vi "Display.vi"(8 "error in":errorcluster, 11 "Plain - Three Button in":refnum<class "Plain - Three Button.lvclass">) -> (0 "error out":errorcluster, 3 "Plain - Three Button out":refnum<class "Plain - Three Button.lvclass">)   [LabVIEW 2021, in "Pop-Up.lvlib" / "Plain - Three Button.lvclass"]
doc: "This is the override method required for each child of the pop up class. It is the pop up that will display to the user.\n\nTo extend this function, create a child class of the pop up class. Then create an override method for this VI. <b>Display.vi</b> is a protected function, therefore it cannot be called in a main application. This VI must be called by a caller function. See one of the standard pop-ups for a setup example.\n\n<b>Code Developed By:</b> +\nDaniel Coons +\nhttps://github.com/danielcoons/tsc-pop-up"
uses:
  Plain - Three Button.lvclass
  C:/Development/Open Source/tsc-pop-up/Popup/Popup.lvclass
  C:/Development/Open Source/tsc-pop-up/Plain/Plain Parent.lvclass
  Popup/Popup.lvclass/Popup.ctl
  Plain Parent.lvclass/Plain Parent.ctl
  Plain - Three Button.lvclass/Plain - Three Button.ctl
  Popup/Data Member Access/Read Theme.vi
  Get Transparent buttons.vi
  Get Dialog Title.vi
  Get Action 1 Text.vi
  Get Action 2 Text.vi
  Get Action 3 Text.vi
  Theme/Theme.lvclass
  Popup/Popup.lvclass
  user32.dll
panel:
  in  "action 3":bool
  in  "action 2":bool
  out "dialog title":string
  out "message":string
  in  "action 1":bool
  # "This VI displays the popup"
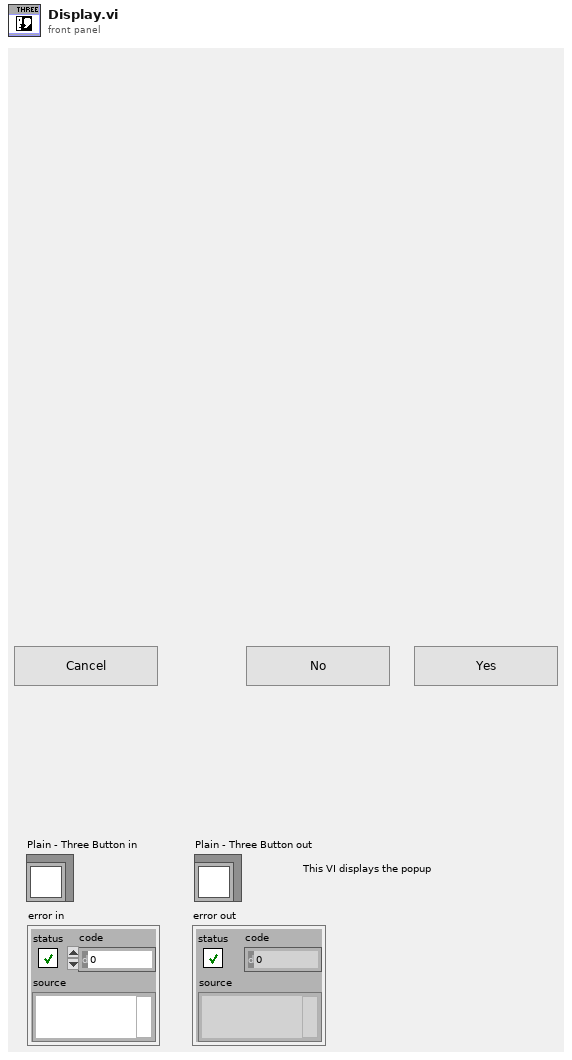
[diagram p1: front panel]
types:
  T1 = typedef "LVRectTypeDef.ctl" = cluster{"Left":i16, "Top":i16, "Right":i16, "Bottom":i16}
  T2 = typedef "LVPointTypeDef.ctl" = cluster{"Horizontal":i16, "Vertical":i16}
  T3 = typedef "LVPoint32TypeDef.ctl" = cluster{"Horizontal":i32, "Vertical":i32}
  T4 = typedef "LVPositionTypeDef.ctl" = cluster{"Left":i32, "Top":i32}
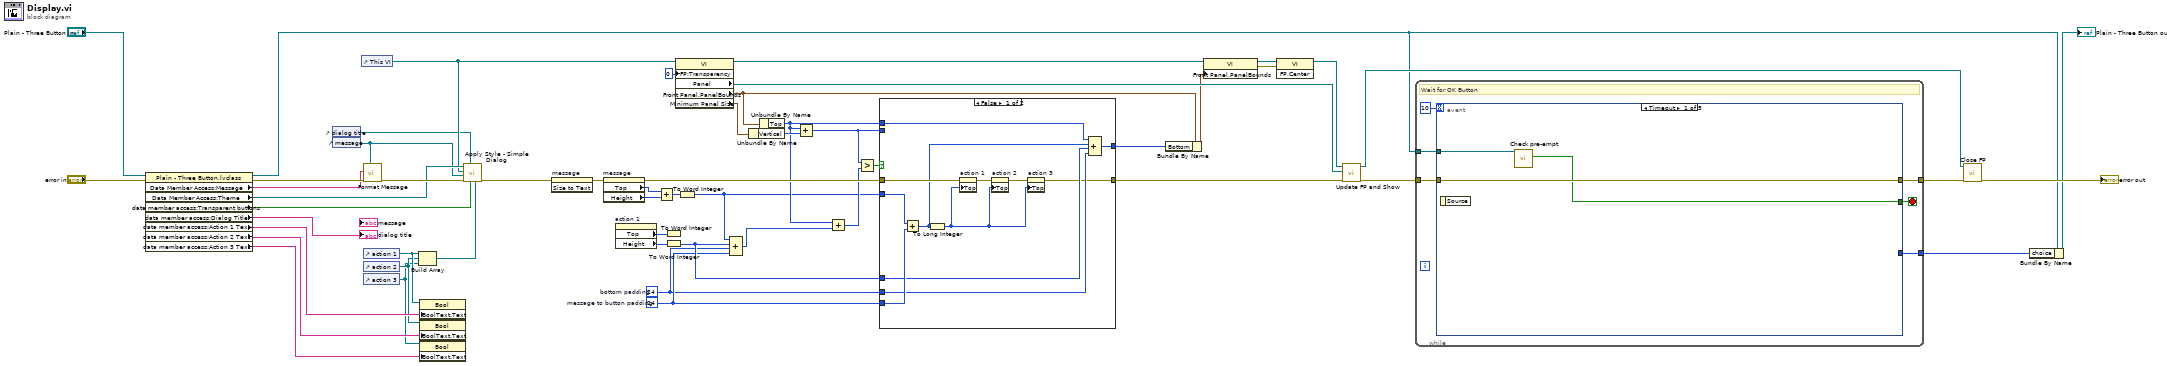
[diagram p0: block diagram]
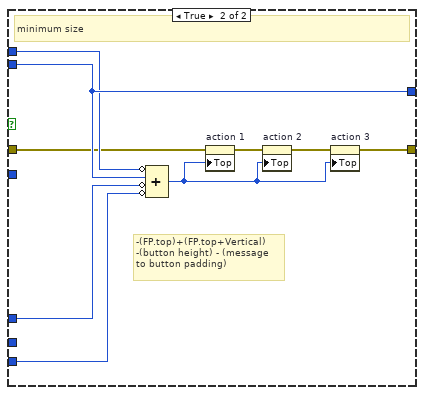
[diagram p2: hidden frame]
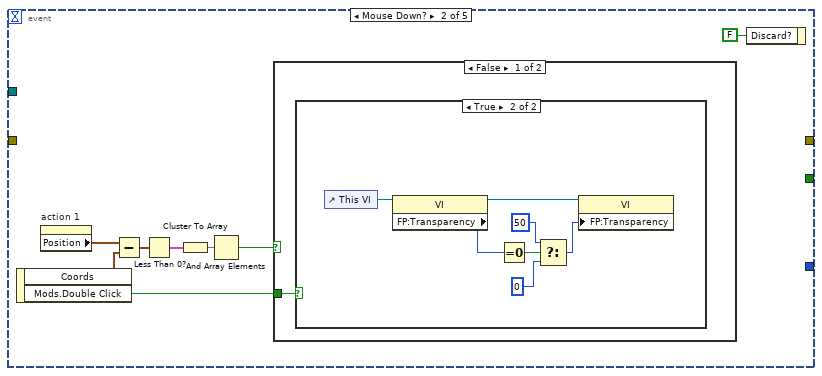
[diagram p3: hidden frame]
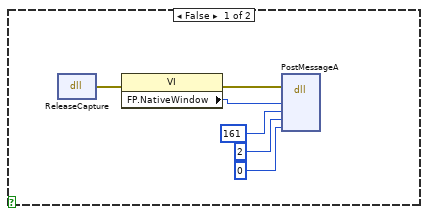
[diagram p4: hidden frame]
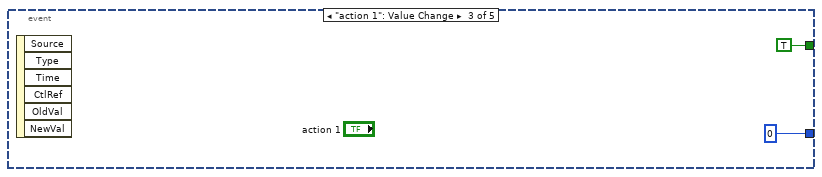
[diagram p6: hidden frame]
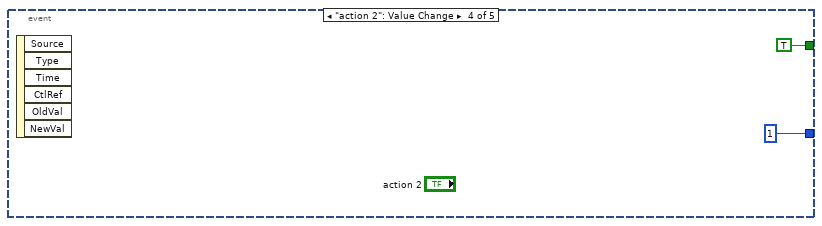
[diagram p7: hidden frame]
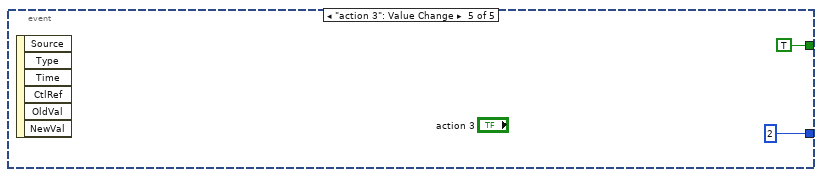
[diagram p8: hidden frame]
diagram:
  w26 = i16 24  # message to button padding
  w24 = i16 24  # bottom padding
  n1 = property class="Plain - Three Button.lvclass"(reference="Plain - Three Button in", error in="error in") -> (reference out=w2:refnum<class "Plain - Three Button.lvclass">, error out=w49:errorcluster, "Data Member Access:Message"=w45:string, "Data Member Access:Theme"=w18:refnum<class "Theme.lvclass">, "data member access:Transparent buttons"=w1:bool, "data member access:Dialog Title"=→"dialog title":string, "data member access:Action 1 Text"=w13:string, "data member access:Action 2 Text"=w12:string, "data member access:Action 3 Text"=w9:string)
  n2 = control-ref of="dialog title"() -> (w5:refnum<vi>)
  n3 = control-ref of="message"() -> (w6:refnum<vi>)
  n4 = control-ref of="This VI"() -> (w17:refnum<vi>)
  n5 = call "Format Message.vi"("formatted string"=w6, "error in"=w49, "String Input"=w45) -> ("error out"=w20:errorcluster)  [unwired: 7 in, 1 out]
  n6 = control-ref of="action 1"() -> (w14:refnum<vi>)
  n7 = control-ref of="action 2"() -> (w11:refnum<vi>)
  n8 = control-ref of="action 3"() -> (w10:refnum<vi>)
  n9 = Build Array(w14, w11, w10) -> (w16:refnum<vi>[])
  n10 = property class="Bool"(reference=w14, "BoolText.Text"=w13) -> ()  [unwired: 1 in, 2 out]
  n11 = property class="Bool"(reference=w11, "BoolText.Text"=w12) -> ()  [unwired: 1 in, 2 out]
  n12 = property class="Bool"(reference=w10, "BoolText.Text"=w9) -> ()  [unwired: 1 in, 2 out]
  n13 = call "Apply Style - Simple Dialog.vi"("button refs"=w16, "keep transparent buttons?"=w1, "title ref"=w5, "error in"=w20, "message ref"=w6, "pop up ref"=w17, "Theme in"=w18) -> ("error out"=w19:errorcluster)  [unwired: 3 in, 1 out]
  n14 = invoke on="message" class="Str" method="Size to Text"(error in=w19) -> (error out=w48:errorcluster)  [unwired: 2 in, 2 out]
  n15 = property on="message" class="Str"(error in=w48) -> (error out=w29:errorcluster, "Top"=w40:i32, "Height"=w39:u32)  [unwired: 1 in, 1 out]
  n16 = property on="action 1" class="Bool"() -> ("Top"=w42:i32, "Height"=w41:u32)  [unwired: 2 in, 2 out]
  n17 = Add(x=w40, y=w39) -> (x+y=w38:u32)
  n18 = To Word Integer(number=w42) -> ()  [unwired: 1 out]
  n19 = To Word Integer(number=w41) -> (16bit integer=w27:i16)
  n20 = property class="VI"(reference=w17, "FP:Transparency"=u8 0 ("Front Panel Window:Transparency")) -> (reference out=w44:refnum<vi>, "Panel"=w43:refnum<vi>, "Front Panel.PanelBounds"=w34:T1, "Minimum Panel Size"=w37:T2)  [unwired: 1 in, 1 out]
  n21 = To Word Integer(number=w38) -> (16bit integer=w3:i16)
  n22 = Compound Arithmetic op=ADD(w3, w27, w24, w26) -> (w4:i16)
  n23 = Unbundle By Name(w37) -> ("Vertical"=w36:i16)
  n24 = Unbundle By Name(w34) -> ("Top"=w21:i16)
  n25 = Add(x=w21, y=w36) -> (x+y=w22:i16)
  n26 = Add(x=w21, y=w4) -> (x+y=w23:i16)
  n27 = Greater?(x=w22, y=w23) -> (0:w30:bool)
  n28 = case shown="False" w30 {
    tunnel: [w65 w75] -> w25
    tunnel: w22 -> [_ w75]
    tunnel: w3 -> [w66 _]
    tunnel: w21 -> [w59 w74]
    tunnel: w29 -> [w64 w73]
    tunnel: [w56 w67] -> w28
    tunnel: w27 -> [w61 w72]
    tunnel: w26 -> [w63 w71]
    tunnel: w24 -> [w62 _]
    frame False {
      n29 = Add(x=w66, y=w63) -> (x+y=w60:i16)
      n30 = To Long Integer(number=w60) -> (32bit integer=w55:i32)
      n31 = property on="action 1" class="Bool"(error in=w64, "Top"=w55) -> (error out=w58:errorcluster)  [unwired: 1 in, 1 out]
      n32 = property on="action 2" class="Bool"(error in=w58, "Top"=w55) -> (error out=w57:errorcluster)  [unwired: 1 in, 1 out]
      n33 = property on="action 3" class="Bool"(error in=w57, "Top"=w55) -> (error out=w56:errorcluster)  [unwired: 1 in, 1 out]
      n34 = Compound Arithmetic op=ADD(w59, w60, w61, w62) -> (w65:i16)
    }
    frame True {
      # "-(FP.top)+(FP.top+Vertical)\n-(button height) - (message\nto button padding)"
      # "minimum size"
      n35 = Compound Arithmetic op=ADD(invert w74, w75, invert w72, invert w71) -> (w68:i16)
      n36 = property on="action 1" class="Bool"(error in=w73, "Top"=w68) -> (error out=w70:errorcluster)  [unwired: 1 in, 1 out]
      n37 = property on="action 2" class="Bool"(error in=w70, "Top"=w68) -> (error out=w69:errorcluster)  [unwired: 1 in, 1 out]
      n38 = property on="action 3" class="Bool"(error in=w69, "Top"=w68) -> (error out=w67:errorcluster)  [unwired: 1 in, 1 out]
    }
  }
  n39 = Bundle By Name(cluster=w34, "Bottom"=w25) -> (w31:T1)
  n40 = property class="VI"(reference=w44, "Front Panel.PanelBounds"=w31) -> (reference out=w35:refnum<vi>, error out=w32:errorcluster)  [unwired: 1 in]
  n41 = invoke class="VI" method="FP.Center"(reference=w35, error in=w32) -> (reference out=w33:refnum<vi>)  [unwired: 1 in, 2 out]
  n42 = call "Update FP and Show.vi"("error in (no error)"=w28, "Panel Ref"=w43, "VI in"=w33) -> ("error out"=w53:errorcluster, "VI out"=w52:refnum<vi>)  [unwired: 7 in]
  n43 = while {
    tunnel: [w79] -> w54
    tunnel: w53 -> [w80]
    tunnel: w2 -> [w77]
    tunnel: [w76] -> w7
    stop <- w81 stop-if-true
    # "Wait for OK Button"
    n44 = event shown="[0] Timeout" {
      selector: _ -> [_ _ _ _ _]
      dyn-events: _ -> [_ _ _ _ _]
      timeout: 10 -> [_ _ _ _ _]
      tunnel: [w82 _ TRUE ("Pre-empted?") TRUE ("Pre-empted?") TRUE ("Pre-empted?")] -> w81
      tunnel: w80 -> [w84 _ _ _ _]
      tunnel: [w84 _ _ _ _] -> w79
      tunnel: w77 -> [w83 _ _ _ _]
      tunnel: [_ _ u8 0 u8 1 u8 2] -> w76
      event Timeout {
        n45 = event-data() -> ()  [unwired: 1 in, 1 out]
        n46 = call "Check pre-empt.vi"("_Popup in"=w83) -> ("Pre-empted?"=w82:bool)  [unwired: 8 in, 2 out]
      }
      event Mouse Down? {
        n47 = event-data() -> ("Coords"=w86:T3, "Mods.Double Click"=w88:bool)  [unwired: 1 in]
        n48 = property on="action 1" class="Bool"() -> ("Position"=w87:T4)  [unwired: 2 in, 2 out]
        n49 = Subtract(x=w87, y=w86) -> (x-y=w89:T4)
        n50 = Less Than 0?(x=w89) -> (x < 0?=w90:cluster{"Left":bool, "Top":bool})
        n51 = Cluster To Array(cluster=w90) -> (array=w91:bool[])
        n52 = And Array Elements(Boolean array=w91) -> (logical AND=w92:bool)
        n53 = case shown="False" w92 {
          tunnel: w88 -> [w93 _]
          frame False {
            n54 = case shown="True" w93 {
              frame False {
                n55 = dll-call lib="user32.dll" fn="ReleaseCapture"() -> (error out=w97:errorcluster)  [unwired: 4 in, 1 out]
                n56 = property class="VI"(error in=w97) -> (error out=w98:errorcluster, "FP.NativeWindow"=w99:u64)  [unwired: 1 in, 1 out]
                n57 = dll-call lib="user32.dll" fn="PostMessageA"(error in=w98, "hWnd"=w99, "Msg"=161, "wParam"=2, "lParam"=0) -> ()  [unwired: 7 in, 2 out]
              }
              frame True {
                n58 = control-ref of="This VI"() -> (w106:refnum<vi>)
                n59 = property class="VI"(reference=w106) -> (reference out=w104:refnum<vi>, "FP:Transparency"=w105:u8)  [unwired: 1 in, 1 out]
                n60 = Equal To 0?(x=w105) -> (x = 0?=w103:bool)
                n61 = Select(t=u8 50, s=w103, f=u8 0) -> (s? t:f=w102:u8)
                n62 = property class="VI"(reference=w104, "FP:Transparency"=w102) -> ()  [unwired: 1 in, 2 out]
              }
            }
          }
          frame True {
          }
        }
        n63 = event-data("Discard?"=FALSE) -> ()  [unwired: 1 in, 1 out]
      }
      event "action 1": Value Change {
        n64 = event-data() -> ()  [unwired: 1 in, 6 out]
      }
      event "action 2": Value Change {
        n65 = event-data() -> ()  [unwired: 1 in, 6 out]
      }
      event "action 3": Value Change {
        n66 = event-data() -> ()  [unwired: 1 in, 6 out]
      }
    }
  }
  n67 = call "Close FP.vi"("error in (no error)"=w54, "VI in"=w52) -> ("error out"=→"error out":errorcluster)  [unwired: 9 in]
  n68 = Bundle By Name(cluster=w2, "choice"=w7) -> (→"Plain - Three Button out":refnum<class "Plain - Three Button.lvclass">)
